vi "ExecuteLineFromScript.vi"(9 "Script in":string, 10 "Console":string, 11 "Queue in":refnum<queue>) -> (3 "Script out":string)   [LabVIEW 2016]
panel:
  out "added":string
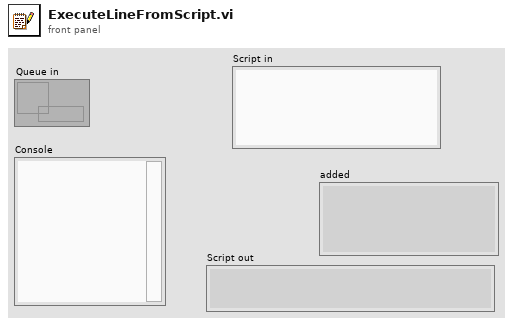
[diagram p1: front panel]
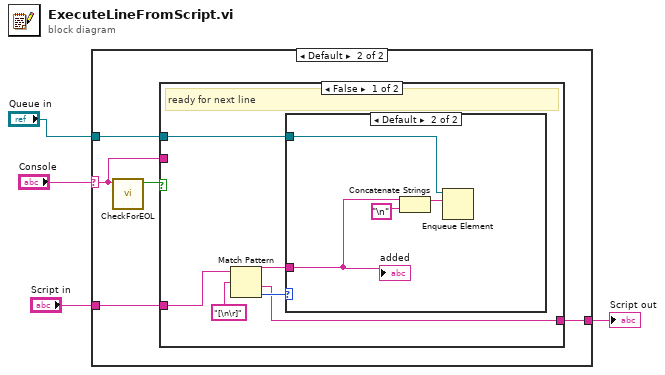
[diagram p0: block diagram]
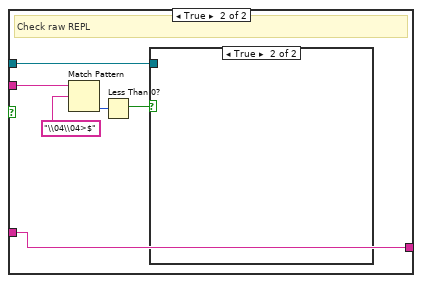
[diagram p4: hidden frame]
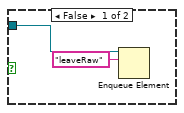
[diagram p5: hidden frame]
diagram:
  n1 = case shown="Default" "Console" {
    selector: "Console" -> [_ w7]
    tunnel: "Script in" -> [w5 w9]
    tunnel: [w5 w8] -> w2
    tunnel: "Queue in" -> [_ w6]
    frame "" {
    }
    frame Default {
      n2 = call "CheckForEOL.vi"("String"=w7) -> ("NOT EOL?"=w10:bool)  [unwired: 10 in]
      n3 = case shown="False" w10 {
        tunnel: w9 -> [w15 w26]
        tunnel: [w13 w26] -> w8
        tunnel: w7 -> [_ w23]
        tunnel: w6 -> [w11 w21]
        frame False {
          # "ready for next line"
          n4 = Match Pattern(string=w15, regular expression="[\n\r]") -> (before substring=w12:string, after substring=w13:string, offset past match=w14:i32)  [unwired: 1 in, 1 out]
          n5 = case shown="Default" w14 {
            tunnel: w12 -> [_ w18]
            tunnel: w11 -> [_ w17]
            frame -1 {
            }
            frame Default {
              n6 = Concatenate Strings(w18, "\n" ("regular expression")) -> (w19:string)
              n7 = Enqueue Element(queue=w17, element=w19) -> ()  [unwired: 2 in, 3 out]
              "added" <- w18
            }
          }
        }
        frame True {
          # "Check raw REPL"
          n8 = Match Pattern(string=w23, regular expression="\\04\\04>$") -> (offset past match=w25:i32)  [unwired: 1 in, 3 out]
          n9 = Less Than 0?(x=w25) -> (x < 0?=w22:bool)
          n10 = case shown="True" w22 {
            tunnel: w21 -> [w28 _]
            frame False {
              n11 = Enqueue Element(queue=w28, element="leaveRaw") -> ()  [unwired: 2 in, 3 out]
            }
            frame True {
            }
          }
        }
      }
    }
  }
  "Script out" <- w2
